vi "To String.vi"(8 "error in (no error)":errorcluster, 11 "JSON Datatype in":refnum<class "JSON Datatype.lvclass">) -> (0 "error out":errorcluster, 3 "String":string)   [LabVIEW 2017, in "LVJSON.lvlib" / "JSON Datatype.lvclass"]
uses:
  JSON Datatype.lvclass
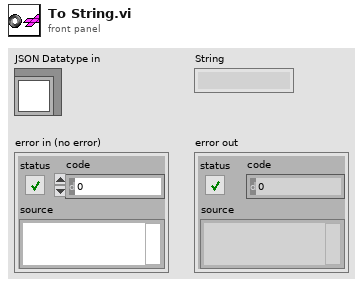
[diagram p1: front panel]
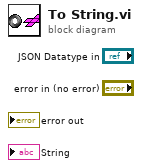
[diagram p0: block diagram]
diagram:
